vi "Query Server Health.vi"(5 "timeout (1000)":i32=1000, 6 "password":string, 7 "Server Address (localhost)":string="localhost", 8 "error in":errorcluster, 9 "username":string, 10 "cookie file":path, 11 "port (8222)":i32=8222) -> (0 "error out":errorcluster, 3 "healthy":bool)   [LabVIEW 2024, in "NATS Infrastructure.lvlib"]
doc: "Checks NATS Server health via http query."
uses:
  NATS Infrastructure.lvlib
  <vilib>/httpClient/LabVIEWHTTPClient.lvlib
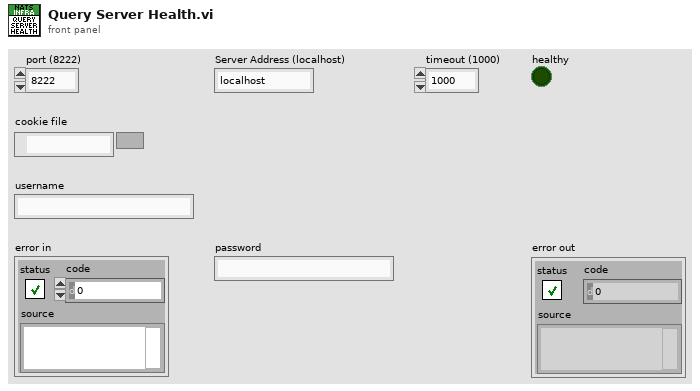
[diagram p1: front panel]
types:
  T1 = typedef "LabVIEWHTTPClient.lvlib/ClientHandle.ctl" = refnum<k1>
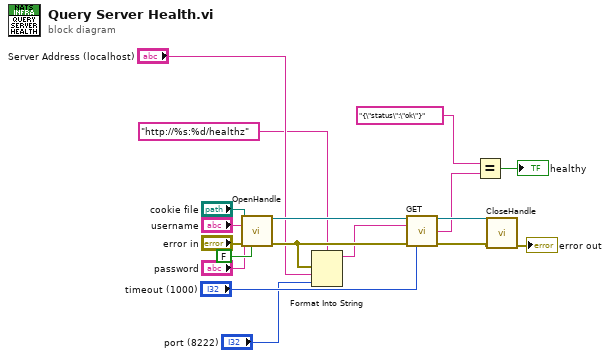
[diagram p0: block diagram]
diagram:
  n1 = call <vilib>:"OpenHandle.vi"("cookie file"="cookie file", "username"="username", "password"="password", "error in (no error)"="error in", "verify server(true)"=FALSE) -> ("client handle out"=w18:T1, "error out"=w5:errorcluster)  [unwired: 9 in]
  n2 = Format Into String(format string="http://%s:%d/healthz" ("url"), error in=w5, "Server Address (localhost)", "port (8222)") -> (resulting string=w2:string)  [unwired: 1 in, 1 out]
  n3 = call <vilib>:"GET.vi"("client handle"=w18, "url"=w2, "error in (no error)"=w5, "timeout (10000)"="timeout (1000)") -> ("client handle out"=w16:T1, "body"=w12:string, "error out"=w15:errorcluster)  [unwired: 8 in, 1 out]
  n4 = Equal?(x="{\"status\":\"ok\"}", y=w12) -> (x = y?=→"healthy":bool)
  n5 = call <vilib>:"CloseHandle.vi"("client handle"=w16, "error in (no error)"=w15) -> ("error out"=→"error out":errorcluster)  [unwired: 13 in]
